vi "Multiple Loops with Notifiers.vi"() -> ()   [LabVIEW 2023]
doc: "This VI demonstrates use of the Messaging Class with notifiers (one-to-many), queues (many-to-one), and User Events. Note that the wire splits but since this is a by-reference scheme, no actual data is copied."
uses:
  Messaging/Messaging.lvclass
panel:
  out "Status":string
  out "From MHL":dbl
  out "FROM EHL":dbl
  in  "Stop":bool
  in  "Data to EHL":dbl
  in  "MHL to EHL":bool
  in  "Data to MHL":dbl
  in  "EHL to MHL":bool
  in  "Start":bool
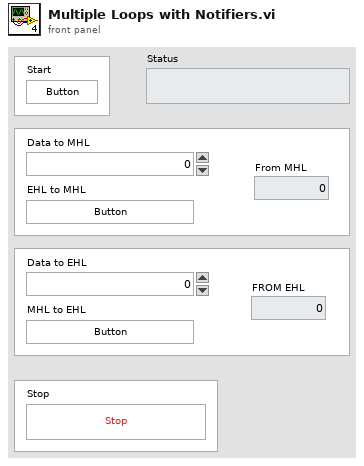
[diagram p1: front panel]
types:
  T1 = typedef "Msg.Event.RegRef.ctl" = refnum<event-registration>
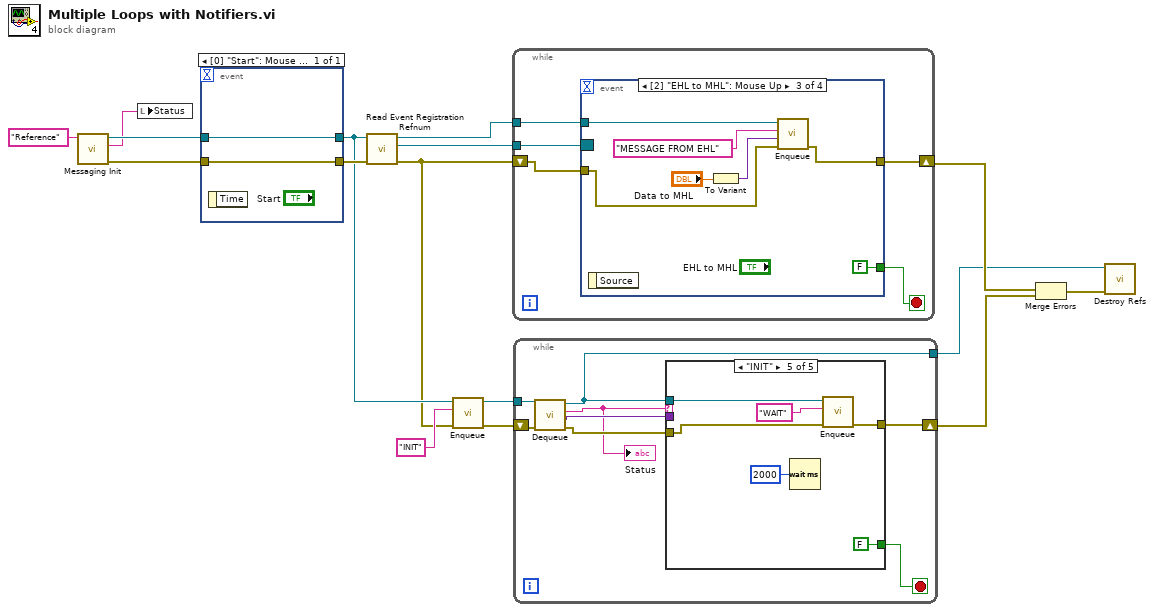
[diagram p0: block diagram]
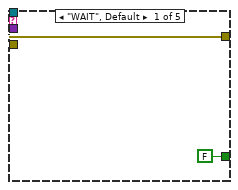
[diagram p2: hidden frame]
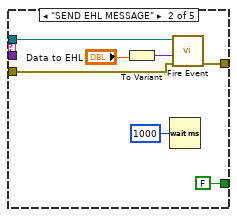
[diagram p3: hidden frame]
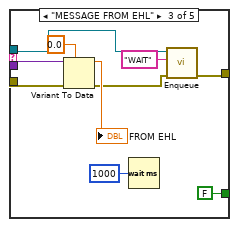
[diagram p4: hidden frame]
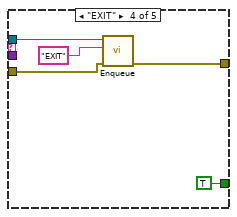
[diagram p5: hidden frame]
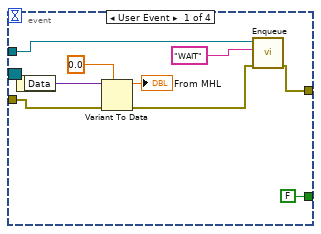
[diagram p6: hidden frame]
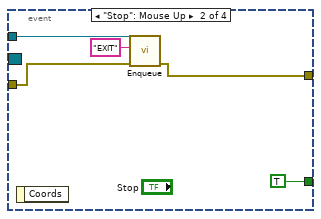
[diagram p7: hidden frame]
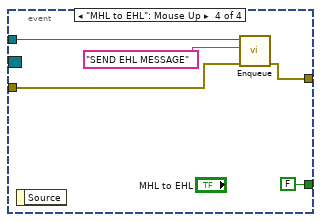
[diagram p8: hidden frame]
diagram:
  n1 = call "Messaging Init.vi"("References Name (in)"="Reference") -> ("error out"=w13:errorcluster, "References Name (out)"=w1:string, "Messaging out"=w15:refnum<class "Messaging.lvclass">)  [unwired: 8 in]
  n2 = local write "Status"(w1) -> ()
  n3 = event shown="[0] \"Start\": Mouse Up" {
    selector: _ -> [_]
    dyn-events: _ -> [_]
    timeout: _ -> [_]
    tunnel: w15 -> [w18]
    tunnel: [w18] -> w10
    tunnel: [w17] -> w14
    tunnel: w13 -> [w17]
    event "Start": Mouse Up {
      n4 = event-data() -> ()  [unwired: 1 in, 1 out]
    }
  }
  n5 = call-dynamic "Read Event Registration Refnum.vi"("error in (no error)"=w14, "Messaging in"=w10) -> ("error out"=w7:errorcluster, "Event Registration Refnum"=w11:T1, "Messaging out"=w12:refnum<class "Messaging.lvclass">)  [unwired: 7 in]
  n6 = call "Enqueue.vi"("error in (no error)"=w7, "Message"="INIT", "Messaging in"=w10) -> ("error out"=w6:errorcluster, "Messaging out"=w8:refnum<class "Messaging.lvclass">)  [unwired: 7 in]
  n7 = while {
    tunnel: w12 -> [w22]
    shift-right: [w20] -> w5
    shift-left: w7 -> [w19]
    tunnel: w11 -> [w23]
    stop <- w21 stop-if-true
    n8 = event shown="[2] \"EHL to MHL\": Mouse Up" {
      selector: w23 -> [_ _ _ _]
      dyn-events: _ -> [_ _ _ _]
      timeout: _ -> [_ _ _ _]
      tunnel: w22 -> [w27 w36 w44 w49]
      tunnel: [FALSE TRUE FALSE FALSE] -> w21
      tunnel: [w24 w33 w39 w45] -> w20
      tunnel: w19 -> [w29 w34 w40 w46]
      event User Event {
        n9 = event-data() -> ("Data"=w32:variant)  [unwired: 1 in]
        n10 = Variant To Data(error in=w29, type=0.0, Variant=w32) -> (data=→"From MHL":dbl, error out=w25:errorcluster)
        n11 = call "Enqueue.vi"("error in (no error)"=w25, "Message"="WAIT", "Messaging in"=w27) -> ("error out"=w24:errorcluster)  [unwired: 7 in, 1 out]
      }
      event "Stop": Mouse Up {
        n12 = event-data() -> ()  [unwired: 1 in, 1 out]
        n13 = call "Enqueue.vi"("error in (no error)"=w34, "Message"="EXIT", "Messaging in"=w36) -> ("error out"=w33:errorcluster)  [unwired: 7 in, 1 out]
      }
      event "EHL to MHL": Mouse Up {
        n14 = event-data() -> ()  [unwired: 1 in, 1 out]
        n15 = To Variant(anything="Data to MHL") -> (Variant=w42:variant)
        n16 = call "Enqueue.vi"("error in (no error)"=w40, "Data"=w42, "Message"="MESSAGE FROM EHL", "Messaging in"=w44) -> ("error out"=w39:errorcluster)  [unwired: 6 in, 1 out]
      }
      event "MHL to EHL": Mouse Up {
        n17 = event-data() -> ()  [unwired: 1 in, 1 out]
        n18 = call "Enqueue.vi"("error in (no error)"=w46, "Message"="SEND EHL MESSAGE", "Messaging in"=w49) -> ("error out"=w45:errorcluster)  [unwired: 7 in, 1 out]
      }
    }
  }
  n19 = while {
    tunnel: w8 -> [w55]
    tunnel: [w50] -> w2
    shift-right: [w56] -> w4
    shift-left: w6 -> [w54]
    stop <- w57 stop-if-true
    n20 = call "Dequeue.vi"("error in (no error)"=w54, "Messaging in"=w55) -> ("error out"=w53:errorcluster, "Data"=w52:variant, "Message"=w51:string, "Messaging out"=w50:refnum<class "Messaging.lvclass">)  [unwired: 6 in]
    "Status" <- w51
    n21 = case shown="\"INIT\"" w51 {
      tunnel: w52 -> [_ _ w76 _ _]
      tunnel: w50 -> [_ w65 w70 w80 w85]
      tunnel: [FALSE FALSE FALSE TRUE FALSE] -> w57
      tunnel: w53 -> [w58 w62 w72 w78 w83]
      tunnel: [w58 w61 w71 w77 w84] -> w56
      frame "WAIT", Default {
      }
      frame "SEND EHL MESSAGE" {
        n22 = To Variant(anything="Data to EHL") -> (Variant=w64:variant)
        n23 = Wait (ms)(milliseconds to wait=u32 1000) -> ()  [unwired: 1 out]
        n24 = call "Fire Event.vi"("error in (no error)"=w62, "Data"=w64, "Messaging in"=w65) -> ("error out"=w61:errorcluster)  [unwired: 7 in, 1 out]
      }
      frame "MESSAGE FROM EHL" {
        n25 = Variant To Data(error in=w72, type=0.0, Variant=w76) -> (data=→"FROM EHL":dbl, error out=w68:errorcluster)
        n26 = Wait (ms)(milliseconds to wait=u32 1000) -> ()  [unwired: 1 out]
        n27 = call "Enqueue.vi"("error in (no error)"=w68, "Message"="WAIT", "Messaging in"=w70) -> ("error out"=w71:errorcluster)  [unwired: 7 in, 1 out]
      }
      frame "EXIT" {
        n28 = call "Enqueue.vi"("error in (no error)"=w78, "Message"="EXIT", "Messaging in"=w80) -> ("error out"=w77:errorcluster)  [unwired: 7 in, 1 out]
      }
      frame "INIT" {
        n29 = Wait (ms)(milliseconds to wait=u32 2000) -> ()  [unwired: 1 out]
        n30 = call "Enqueue.vi"("error in (no error)"=w83, "Message"="WAIT", "Messaging in"=w85) -> ("error out"=w84:errorcluster)  [unwired: 7 in, 1 out]
      }
    }
  }
  n31 = Merge Errors(w5, w4) -> (w3:errorcluster)
  n32 = call "Destroy Refs.vi"("error in (no error)"=w3, "Messaging in"=w2) -> ()  [unwired: 9 in, 1 out]
